vi "Read Process Variable.vi"(8 "error in (no error)":errorcluster, 11 "PID Loop in":refnum<class "PID Loop.lvclass">) -> (0 "error out":errorcluster, 2 "process variable":dbl, 3 "PID Loop out":refnum<class "PID Loop.lvclass">)   [LabVIEW 2024]
uses:
  PID Loop.lvclass
  PID Loop.lvclass/PID Loop.ctl
  C:/Users/uspoaotto/OneDrive - Oregon Tool/Desktop/working copies/zeroTimeoutMessageHandler/src/Zero Timeout Message Handler/Zero Timeout Message Handler/Zero Timeout Message Handler.lvclass
  C:/Users/uspoaotto/OneDrive - Oregon Tool/Desktop/working copies/zeroTimeoutMessageHandler/samples/PID Controller/PID Loop/PID Loop/PID Loop.lvclass
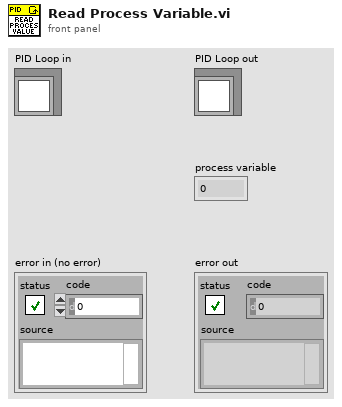
[diagram p1: front panel]
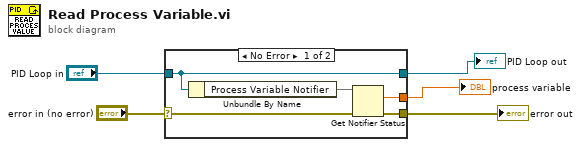
[diagram p0: block diagram]
diagram:
  n1 = case shown="No Error" "error in (no error)" {
    selector: "error in (no error)" -> [w8 w12]
    tunnel: [w7 w12] -> w4
    tunnel: [w10 w11] -> w2
    tunnel: "PID Loop in" -> [w10 w11]
    tunnel: [w6 _] -> w1
    frame No Error {
      n2 = Unbundle By Name(w10) -> ("Process Variable Notifier"=w9)
      n3 = Get Notifier Status(notifier=w9, error in (no error)=w8) -> (current notification=w6:dbl, error out=w7:errorcluster)  [unwired: 3 out]
    }
    frame Error {
    }
  }
  "error out" <- w4
  "PID Loop out" <- w2
  "process variable" <- w1
